vi "新版加标流程.vi"(8 "error in (no error)":errorcluster caption="错误输入（无错误）", 11 "参数":enum16{"氨氮", "总磷", "总氮", "CODMn", "CODcr"}(ring)) -> (0 "error out":errorcluster caption="错误输出")   [LabVIEW 2016, in "质控单元.lvlib"]
panel:
  out "Next State":string
  out "数值":i32
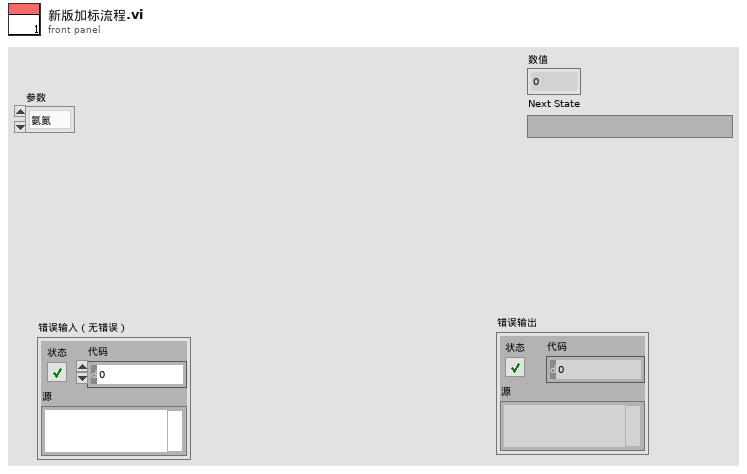
[diagram p1: front panel]
types:
  T1 = cluster{"时间标识":timestamp, "设备":string, "日志信息":string}
  T2 = enum16{"待机", "润洗中", "进样中", "加标中", "排液中", "搅拌中", "进样超时报警"}
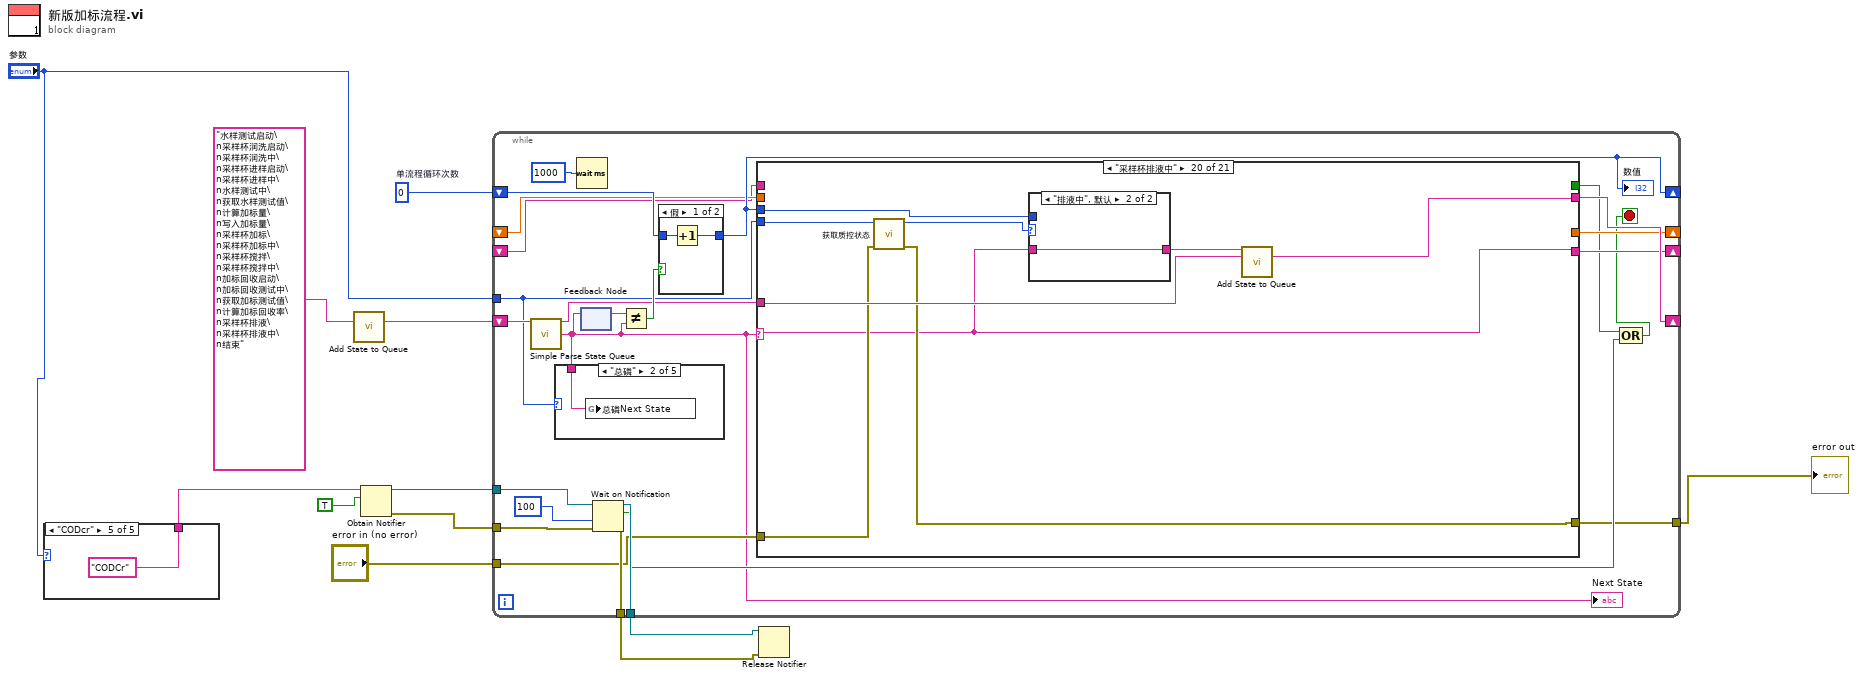
[diagram p0: block diagram]
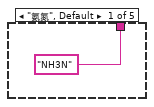
[diagram p2: hidden frame]
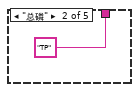
[diagram p3: hidden frame]
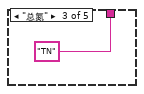
[diagram p4: hidden frame]
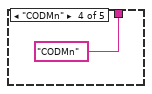
[diagram p5: hidden frame]
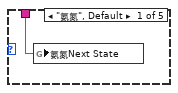
[diagram p6: hidden frame]
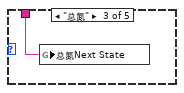
[diagram p7: hidden frame]
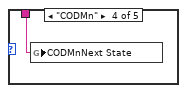
[diagram p8: hidden frame]
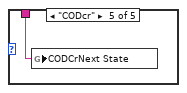
[diagram p9: hidden frame]
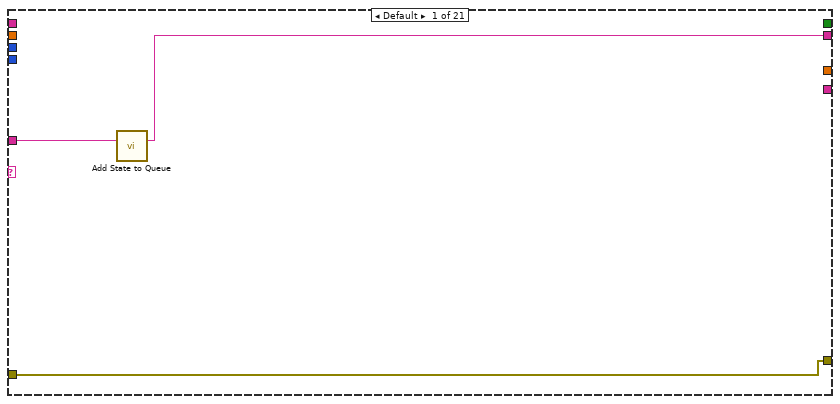
[diagram p11: hidden frame]
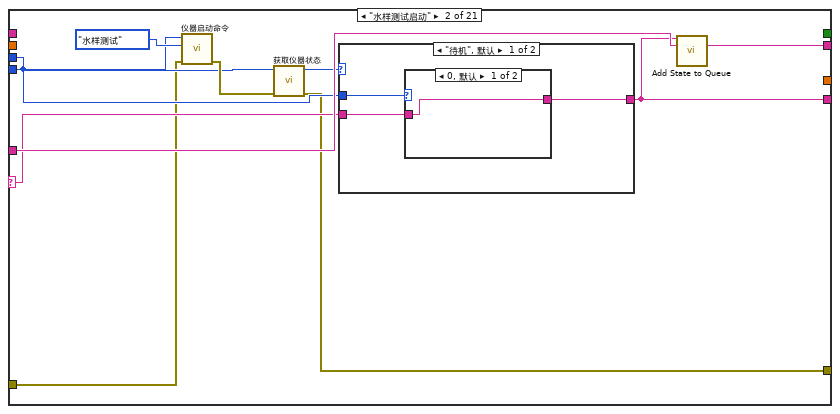
[diagram p12: hidden frame]
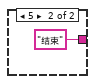
[diagram p13: hidden frame]
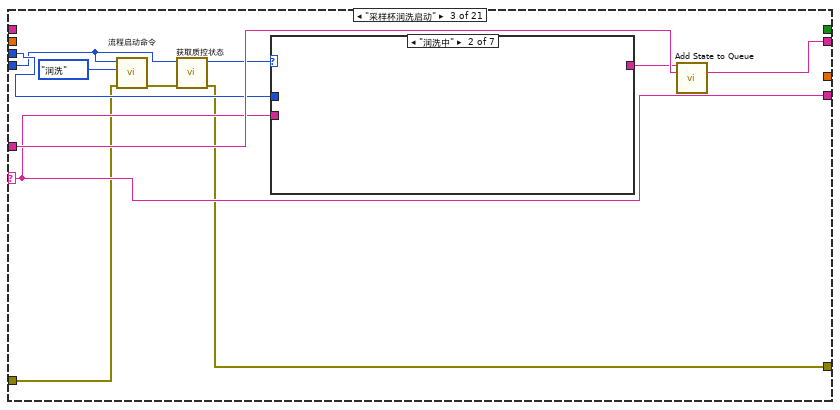
[diagram p15: hidden frame]
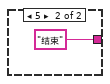
[diagram p17: hidden frame]
diagram:
  w10 = 0  # 单流程循环次数
  n1 = case shown="\"CODcr\"" "参数" {
    tunnel: ["NH3N" ("名称（未命名）") "TP" ("名称（未命名）") "TN" ("名称（未命名）") "CODMn" ("名称（未命名）") "CODCr" ("名称（未命名）")] -> w4
    frame "氨氮", Default {
    }
    frame "总磷" {
    }
    frame "总氮" {
    }
    frame "CODMn" {
    }
    frame "CODcr" {
    }
  }
  n2 = call "Add State to Queue.vi"("State(s) In (\"\")"="水样测试启动\n采样杯润洗启动\n采样杯润洗中\n采样杯进样启动\n采样杯进样中\n水样测试中\n获取水样测试值\n计算加标量\n写入加标量\n采样杯加标\n采样杯加标中\n采样杯搅拌\n采样杯搅拌中\n加标回收启动\n加标回收测试中\n获取加标测试值\n计算加标回收率\n采样杯排液\n采样杯排液中\n结束" ("State(s) In (\"\")")) -> ("States Out"=w11:string)  [unwired: 14 in]
  n3 = Obtain Notifier(name (unnamed)=w4, notification data type=TRUE) -> (notifier out=w6:refnum<notifier>, error out=w5:errorcluster)  [unwired: 2 in, 1 out]
  n4 = while {
    shift-right: [w40] -> _
    shift-left: w11 -> [w41]
    tunnel: "参数" -> [w19]
    shift-right: [w36] -> _
    shift-left: w10 -> [w37]
    shift-right: [w34] -> _
    shift-left: _ -> [w33]
    shift-right: [w32] -> _
    shift-left: _ -> [w31]
    tunnel: [w21] -> w8
    tunnel: "error in (no error)" -> [w20]
    tunnel: w6 -> [w29]
    tunnel: w5 -> [w28]
    tunnel: [w27] -> w2
    tunnel: [w26] -> w1
    stop <- w23 stop-if-true
    n5 = call "Simple Parse State Queue.vi"("State Queue"=w41) -> ("Remain States"=w22:string, "Next State"=w18:string)  [unwired: 13 in]
    "Next State" <- w18
    n6 = case shown="\"总磷\"" w19 {
      tunnel: w18 -> [w42 w43 w44 w45 w46]
      frame "氨氮", Default {
        n7 = global write "质控内部交互全局.vi" "氨氮Next State"(w42) -> ()
      }
      frame "总磷" {
        n8 = global write "质控内部交互全局.vi" "总磷Next State"(w43) -> ()
      }
      frame "总氮" {
        n9 = global write "质控内部交互全局.vi" "总氮Next State"(w44) -> ()
      }
      frame "CODMn" {
        n10 = global write "质控内部交互全局.vi" "CODMnNext State"(w45) -> ()
      }
      frame "CODcr" {
        n11 = global write "质控内部交互全局.vi" "CODCrNext State"(w46) -> ()
      }
    }
    n12 = Wait (ms)(milliseconds to wait=u32 1000 ("等待时间（毫秒）")) -> ()  [unwired: 1 out]
    n13 = feedback-in #1(w18) -> ()
    n14 = feedback #1() -> (w39:string)  [unwired: 1 in]
    n15 = Wait on Notification(notifier=w29, timeout in ms (-1)=100 ("超时毫秒(-1)"), error in (no error)=w28) -> (notifier out=w27:refnum<notifier>, notification=w24:bool, error out=w26:errorcluster)  [unwired: 1 in, 1 out]
    n16 = Not Equal?(x=w39, y=w18) -> (x != y?=w38:bool)
    n17 = case shown="假" w38 {
      tunnel: w37 -> [w48 _]
      tunnel: [w47 _] -> w36
      frame False {
        n18 = Increment(x=w48) -> (x+1=w47:i32)
      }
      frame True {
      }
    }
    "数值" <- w36
    n19 = case shown="\"采样杯排液中\"" w18 {
      selector: w18 -> [_ w56 w70 w88 w99 w115 w127 w136 w145 w159 w173 w185 w195 w207 w217 w233 w243 w254 w264 w277 w295]
      tunnel: w22 -> [w51 w61 w78 w93 w106 w121 w132 w141 w151 w165 w181 w191 w203 w211 w225 w239 w248 w257 w268 w281 w290]
      tunnel: [w50 w60 w77 w92 w105 w120 w131 w140 w150 w164 w180 w190 w202 w209 w224 w238 w247 w256 w265 w278 w297] -> w40
      tunnel: w19 -> [_ w58 w74 w90 w102 w117 w130 w139 w148 w162 w177 w188 w198 w210 w220 w237 w246 w252 w269 w282 w291]
      tunnel: w36 -> [_ w57 w76 w91 w104 w118 w129 w138 w149 w163 w179 w189 w201 w212 w223 w236 w245 w255 w270 w283 w296]
      tunnel: [_ _ _ _ _ _ _ _ _ _ _ _ _ _ _ _ _ _ _ _ TRUE] -> w25
      tunnel: [_ _ _ _ _ _ _ _ w147 _ _ _ _ _ _ _ _ _ _ _ _] -> w34
      tunnel: w33 -> [_ _ _ _ _ _ _ _ _ w161 _ _ _ _ _ _ _ _ _ _ _]
      tunnel: [_ w54 w70 w88 w99 w115 w127 w136 w145 w159 w173 w185 w195 w207 w217 w233 w243 w251 w264 w277 _] -> w32
      tunnel: w31 -> [_ _ _ _ _ _ _ _ _ _ _ _ _ _ _ _ _ _ _ _ w289]
      tunnel: [w49 w53 w69 w87 w97 w113 w125 w135 w143 w158 w172 w184 w194 w206 w216 w231 w242 w250 w266 w279 w286] -> w21
      tunnel: w20 -> [w49 w52 w68 w86 w96 w116 w124 w134 w144 w157 w171 w183 w193 w205 w215 w232 w241 w250 w267 w280 w286]
      frame Default {
        n20 = call "Add State to Queue.vi"("State(s) In (\"\")"=w51) -> ("States Out"=w50:string)  [unwired: 14 in]
      }
      frame "水样测试启动" {
        n21 = call "仪器启动命令.vi"("error in (no error)"=w52, "测试模式"=enum16{"水样测试", "加标回收"}."水样测试", "参数"=w58) -> ("error out"=w59:errorcluster)  [unwired: 8 in]
        n22 = call "获取仪器状态.vi"("error in (no error)"=w59, "参数"=w58) -> ("error out"=w53:errorcluster, "仪器状态"=w55:enum16{"待机", "运行"})  [unwired: 8 in]
        n23 = case shown="\"待机\", 默认" w55 {
          tunnel: w57 -> [w65 _]
          tunnel: w56 -> [w64 _]
          tunnel: [w63 _] -> w54
          frame "待机", Default {
            n24 = case shown="0, 默认" w65 {
              tunnel: w64 -> [w66 _]
              tunnel: [w66 "结束"] -> w63
              frame 0, Default {
              }
              frame 5 {
              }
            }
          }
          frame "运行" {
          }
        }
        n25 = call "Add State to Queue.vi"("State(s) In Front (\"\")"=w54, "State(s) In (\"\")"=w61) -> ("States Out"=w60:string)  [unwired: 13 in]
      }
      frame "采样杯润洗启动" {
        n26 = call "流程启动命令.vi"("error in (no error)"=w68, "流程"=enum16{"润洗", "进样", "加标", "搅拌", "排液"}."润洗", "参数"=w74) -> ("error out"=w72:errorcluster)  [unwired: 8 in]
        n27 = call "获取质控状态.vi"("error in (no error)"=w72, "参数"=w74) -> ("error out"=w69:errorcluster, "仪器状态"=w73:T2)  [unwired: 8 in]
        n28 = case shown="\"润洗中\"" w73 {
          tunnel: w76 -> [w81 _ _ _ _ _ _]
          tunnel: w70 -> [w80 _ _ _ _ _ _]
          tunnel: [w79 _ _ _ _ _ "结束"] -> w71
          frame "待机", Default {
            n29 = case shown="0, 默认" w81 {
              tunnel: w80 -> [w82 _]
              tunnel: [w82 "结束"] -> w79
              frame 0, Default {
              }
              frame 5 {
              }
            }
          }
          frame "润洗中" {
          }
          frame "进样中" {
          }
          frame "加标中" {
          }
          frame "排液中" {
          }
          frame "搅拌中" {
          }
          frame "进样超时报警" {
          }
        }
        n30 = call "Add State to Queue.vi"("State(s) In Front (\"\")"=w71, "State(s) In (\"\")"=w78) -> ("States Out"=w77:string)  [unwired: 13 in]
      }
      frame "采样杯润洗中" {
        n31 = call "获取质控状态.vi"("error in (no error)"=w86, "参数"=w90) -> ("error out"=w87:errorcluster, "仪器状态"=w85:T2)  [unwired: 8 in]
        n32 = case shown="\"润洗中\", 默认" w85 {
          tunnel: w91 -> [_ _ _]
          tunnel: w88 -> [_ w94 _]
          tunnel: [_ w94 "结束"] -> w89
          frame "待机" {
          }
          frame "润洗中", Default {
          }
          frame "进样超时报警" {
          }
        }
        n33 = call "Add State to Queue.vi"("State(s) In Front (\"\")"=w89, "State(s) In (\"\")"=w93) -> ("States Out"=w92:string)  [unwired: 13 in]
      }
      frame "采样杯进样启动" {
        n34 = call "流程启动命令.vi"("error in (no error)"=w96, "流程"=enum16{"润洗", "进样", "加标", "搅拌", "排液"}."进样", "参数"=w102) -> ("error out"=w98:errorcluster)  [unwired: 8 in]
        n35 = call "获取质控状态.vi"("error in (no error)"=w98, "参数"=w102) -> ("error out"=w97:errorcluster, "仪器状态"=w101:T2)  [unwired: 8 in]
        n36 = case shown="\"待机\", 默认" w101 {
          tunnel: w104 -> [w109 _ _]
          tunnel: w99 -> [w108 _ _]
          tunnel: [w107 _ "结束"] -> w100
          frame "待机", Default {
            n37 = case shown="0, 默认" w109 {
              tunnel: w108 -> [w110 _]
              tunnel: [w110 "结束"] -> w107
              frame 0, Default {
              }
              frame 5 {
              }
            }
          }
          frame "进样中" {
          }
          frame "进样超时报警" {
          }
        }
        n38 = call "Add State to Queue.vi"("State(s) In Front (\"\")"=w100, "State(s) In (\"\")"=w106) -> ("States Out"=w105:string)  [unwired: 13 in]
      }
      frame "采样杯进样中" {
        n39 = call "获取质控状态.vi"("error in (no error)"=w116, "参数"=w117) -> ("error out"=w113:errorcluster, "仪器状态"=w119:T2)  [unwired: 8 in]
        n40 = case shown="\"进样中\", 默认" w119 {
          tunnel: w118 -> [_ _ _]
          tunnel: w115 -> [_ w122 _]
          tunnel: [_ w122 "结束"] -> w114
          frame "待机" {
          }
          frame "进样中", Default {
          }
          frame "进样超时报警" {
          }
        }
        n41 = call "Add State to Queue.vi"("State(s) In Front (\"\")"=w114, "State(s) In (\"\")"=w121) -> ("States Out"=w120:string)  [unwired: 13 in]
      }
      frame "水样测试中" {
        n42 = call "获取仪器状态.vi"("error in (no error)"=w124, "参数"=w130) -> ("error out"=w125:errorcluster, "仪器状态"=w128:enum16{"待机", "运行"})  [unwired: 8 in]
        n43 = case shown="\"待机\"" w128 {
          tunnel: w129 -> [_ _]
          tunnel: w127 -> [_ w133]
          tunnel: [_ w133] -> w126
          frame "待机" {
          }
          frame "运行", Default {
          }
        }
        n44 = call "Add State to Queue.vi"("State(s) In Front (\"\")"=w126, "State(s) In (\"\")"=w132) -> ("States Out"=w131:string)  [unwired: 13 in]
      }
      frame "获取水样测试值" {
        n45 = call "获取仪器状态.vi"("error in (no error)"=w134, "参数"=w139) -> ("error out"=w135:errorcluster)  [unwired: 8 in, 1 out]
        n46 = case shown="0, 默认" w138 {
          tunnel: w136 -> [w142 _]
          tunnel: [w142 _] -> w137
          frame 0, Default {
          }
          frame 5 {
          }
        }
        n47 = call "Add State to Queue.vi"("State(s) In Front (\"\")"=w137, "State(s) In (\"\")"=w141) -> ("States Out"=w140:string)  [unwired: 13 in]
      }
      frame "计算加标量" {
        n48 = call "计算加标体积.vi"("error in (no error)"=w144, "参数"=w148) -> ("error out"=w143:errorcluster, "加标体积"=w147:dbl)  [unwired: 7 in, 1 out]
        n49 = case shown="错误" w143 {
          tunnel: w149 -> [_ w154]
          tunnel: w145 -> [_ w153]
          tunnel: [_ w152] -> w146
          frame No Error {
          }
          frame Error {
            n50 = case shown="5" w154 {
              tunnel: w153 -> [w155 _]
              tunnel: [w155 "结束"] -> w152
              frame 0, Default {
              }
              frame 5 {
              }
            }
          }
        }
        n51 = call "Add State to Queue.vi"("State(s) In Front (\"\")"=w146, "State(s) In (\"\")"=w151) -> ("States Out"=w150:string)  [unwired: 13 in]
      }
      frame "写入加标量" {
        n52 = call "写入加标体积.vi"("加标体积"=w161, "error in (no error)"=w157, "参数"=w162) -> ("error out"=w158:errorcluster)  [unwired: 8 in]
        n53 = case shown="错误" w158 {
          tunnel: w163 -> [_ w168]
          tunnel: w159 -> [_ w167]
          tunnel: [_ w166] -> w160
          frame No Error {
          }
          frame Error {
            n54 = case shown="5" w168 {
              tunnel: w167 -> [w169 _]
              tunnel: [w169 "结束"] -> w166
              frame 0, Default {
              }
              frame 5 {
              }
            }
          }
        }
        n55 = call "Add State to Queue.vi"("State(s) In Front (\"\")"=w160, "State(s) In (\"\")"=w165) -> ("States Out"=w164:string)  [unwired: 13 in]
      }
      frame "采样杯加标" {
        n56 = call "流程启动命令.vi"("error in (no error)"=w171, "流程"=enum16{"润洗", "进样", "加标", "搅拌", "排液"}."加标", "参数"=w177) -> ("error out"=w176:errorcluster)  [unwired: 8 in]
        n57 = call "获取质控状态.vi"("error in (no error)"=w176, "参数"=w177) -> ("error out"=w172:errorcluster, "仪器状态"=w175:T2)  [unwired: 8 in]
        n58 = case shown="\"待机\", 默认" w175 {
          tunnel: w179 -> [_ _]
          tunnel: w173 -> [w182 _]
          tunnel: [w182 _] -> w174
          frame "待机", Default {
          }
          frame "加标中" {
          }
        }
        n59 = call "Add State to Queue.vi"("State(s) In Front (\"\")"=w174, "State(s) In (\"\")"=w181) -> ("States Out"=w180:string)  [unwired: 13 in]
      }
      frame "采样杯加标中" {
        n60 = call "获取质控状态.vi"("error in (no error)"=w183, "参数"=w188) -> ("error out"=w184:errorcluster, "仪器状态"=w187:T2)  [unwired: 8 in]
        n61 = case shown="\"加标中\", 默认" w187 {
          tunnel: w189 -> [_ _]
          tunnel: w185 -> [_ w192]
          tunnel: [_ w192] -> w186
          frame "待机" {
          }
          frame "加标中", Default {
          }
        }
        n62 = call "Add State to Queue.vi"("State(s) In Front (\"\")"=w186, "State(s) In (\"\")"=w191) -> ("States Out"=w190:string)  [unwired: 13 in]
      }
      frame "采样杯搅拌" {
        n63 = call "流程启动命令.vi"("error in (no error)"=w193, "流程"=enum16{"润洗", "进样", "加标", "搅拌", "排液"}."搅拌", "参数"=w198) -> ("error out"=w199:errorcluster)  [unwired: 8 in]
        n64 = call "获取质控状态.vi"("error in (no error)"=w199, "参数"=w198) -> ("error out"=w194:errorcluster, "仪器状态"=w197:T2)  [unwired: 8 in]
        n65 = case shown="\"搅拌中\"" w197 {
          tunnel: w201 -> [_ _]
          tunnel: w195 -> [w204 _]
          tunnel: [w204 _] -> w196
          frame "待机", Default {
          }
          frame "搅拌中" {
          }
        }
        n66 = call "Add State to Queue.vi"("State(s) In Front (\"\")"=w196, "State(s) In (\"\")"=w203) -> ("States Out"=w202:string)  [unwired: 13 in]
      }
      frame "采样杯搅拌中" {
        n67 = call "获取质控状态.vi"("error in (no error)"=w205, "参数"=w210) -> ("error out"=w206:errorcluster, "仪器状态"=w213:T2)  [unwired: 8 in]
        n68 = case shown="\"搅拌中\", 默认" w213 {
          tunnel: w212 -> [_ _]
          tunnel: w207 -> [_ w214]
          tunnel: [_ w214] -> w208
          frame "待机" {
          }
          frame "搅拌中", Default {
          }
        }
        n69 = call "Add State to Queue.vi"("State(s) In Front (\"\")"=w208, "State(s) In (\"\")"=w211) -> ("States Out"=w209:string)  [unwired: 13 in]
      }
      frame "加标回收启动" {
        n70 = call "仪器启动命令.vi"("error in (no error)"=w215, "测试模式"=enum16{"水样测试", "加标回收"}."加标回收", "参数"=w220) -> ("error out"=w221:errorcluster)  [unwired: 8 in]
        n71 = call "获取仪器状态.vi"("error in (no error)"=w221, "参数"=w220) -> ("error out"=w216:errorcluster, "仪器状态"=w219:enum16{"待机", "运行"})  [unwired: 8 in]
        n72 = case shown="\"待机\", 默认" w219 {
          tunnel: w223 -> [w228 _]
          tunnel: w217 -> [w227 _]
          tunnel: [w226 _] -> w218
          frame "待机", Default {
            n73 = case shown="5" w228 {
              tunnel: w227 -> [w229 _]
              tunnel: [w229 "结束"] -> w226
              frame 0, Default {
              }
              frame 5 {
              }
            }
          }
          frame "运行" {
          }
        }
        n74 = call "Add State to Queue.vi"("State(s) In Front (\"\")"=w218, "State(s) In (\"\")"=w225) -> ("States Out"=w224:string)  [unwired: 13 in]
      }
      frame "加标回收测试中" {
        n75 = call "获取仪器状态.vi"("error in (no error)"=w232, "参数"=w237) -> ("error out"=w231:errorcluster, "仪器状态"=w235:enum16{"待机", "运行"})  [unwired: 8 in]
        n76 = case shown="\"运行\"" w235 {
          tunnel: w236 -> [_ _]
          tunnel: w233 -> [_ w240]
          tunnel: [_ w240] -> w234
          frame "待机", Default {
          }
          frame "运行" {
          }
        }
        n77 = call "Add State to Queue.vi"("State(s) In Front (\"\")"=w234, "State(s) In (\"\")"=w239) -> ("States Out"=w238:string)  [unwired: 13 in]
      }
      frame "获取加标测试值" {
        n78 = call "获取仪器状态.vi"("error in (no error)"=w241, "参数"=w246) -> ("error out"=w242:errorcluster)  [unwired: 8 in, 1 out]
        n79 = case shown="0, 默认" w245 {
          tunnel: w243 -> [w249 _]
          tunnel: [w249 _] -> w244
          frame 0, Default {
          }
          frame 5 {
          }
        }
        n80 = call "Add State to Queue.vi"("State(s) In Front (\"\")"=w244, "State(s) In (\"\")"=w248) -> ("States Out"=w247:string)  [unwired: 13 in]
      }
      frame "计算加标回收率" {
        n81 = case shown="5" w255 {
          tunnel: w254 -> [w263 _]
          tunnel: [w263 _] -> w251
          frame 0, Default {
          }
          frame 5 {
          }
        }
        n82 = case shown="\"总磷\"" w252 {
          tunnel: TRUE ("氨氮加标回收测完标志") -> [w258 w259 w260 w261 w262]
          frame "氨氮", Default {
            n83 = global write "质控测完标志全局 1.vi" "氨氮加标回收测完标志"(w258) -> ()
          }
          frame "总磷" {
            n84 = global write "质控测完标志全局 1.vi" "总磷加标回收测完标志"(w259) -> ()
          }
          frame "总氮" {
            n85 = global write "质控测完标志全局 1.vi" "总氮加标回收测完标志"(w260) -> ()
          }
          frame "CODMn" {
            n86 = global write "质控测完标志全局 1.vi" "COD加标回收测完标志"(w261) -> ()
          }
          frame "CODcr" {
            n87 = global write "质控测完标志全局 1.vi" "CODCr加标回收测完标志"(w262) -> ()
          }
        }
        n88 = call "Add State to Queue.vi"("State(s) In Front (\"\")"=w251, "State(s) In (\"\")"=w257) -> ("States Out"=w256:string)  [unwired: 13 in]
      }
      frame "采样杯排液" {
        n89 = call "流程启动命令.vi"("error in (no error)"=w267, "流程"=enum16{"润洗", "进样", "加标", "搅拌", "排液"}."排液", "参数"=w269) -> ("error out"=w273:errorcluster)  [unwired: 8 in]
        n90 = call "获取质控状态.vi"("error in (no error)"=w273, "参数"=w269) -> ("error out"=w266:errorcluster, "仪器状态"=w272:T2)  [unwired: 8 in]
        n91 = case shown="\"排液中\"" w272 {
          tunnel: w270 -> [_ _]
          tunnel: w264 -> [w275 _]
          tunnel: [w275 _] -> w271
          frame "待机", Default {
          }
          frame "排液中" {
          }
        }
        n92 = call "Add State to Queue.vi"("State(s) In Front (\"\")"=w271, "State(s) In (\"\")"=w268) -> ("States Out"=w265:string)  [unwired: 13 in]
      }
      frame "采样杯排液中" {
        n93 = call "获取质控状态.vi"("error in (no error)"=w280, "参数"=w282) -> ("error out"=w279:errorcluster, "仪器状态"=w276:T2)  [unwired: 8 in]
        n94 = case shown="\"排液中\", 默认" w276 {
          tunnel: w283 -> [_ _]
          tunnel: w277 -> [_ w285]
          tunnel: [_ w285] -> w284
          frame "待机" {
          }
          frame "排液中", Default {
          }
        }
        n95 = call "Add State to Queue.vi"("State(s) In Front (\"\")"=w284, "State(s) In (\"\")"=w281) -> ("States Out"=w278:string)  [unwired: 13 in]
      }
      frame "结束" {
        n96 = call "获取仪器状态.vi"("参数"=w291) -> ()  [unwired: 9 in, 2 out]
        n97 = case shown="0, 默认" w296 {
          tunnel: w295 -> [w310 _]
          tunnel: [w310 _] -> w294
          frame 0, Default {
          }
          frame 5 {
          }
        }
        n98 = case shown="\"氨氮\", 默认" w291 {
          tunnel: FALSE ("氨氮加标回收测完标志") -> [w305 w306 w307 w308 w309]
          frame "氨氮", Default {
            n99 = global write "质控测完标志全局 1.vi" "氨氮加标回收测完标志"(w305) -> ()
          }
          frame "总磷" {
            n100 = global write "质控测完标志全局 1.vi" "总磷加标回收测完标志"(w306) -> ()
          }
          frame "总氮" {
            n101 = global write "质控测完标志全局 1.vi" "总氮加标回收测完标志"(w307) -> ()
          }
          frame "CODMn" {
            n102 = global write "质控测完标志全局 1.vi" "COD加标回收测完标志"(w308) -> ()
          }
          frame "CODcr" {
            n103 = global write "质控测完标志全局 1.vi" "CODCr加标回收测完标志"(w309) -> ()
          }
        }
        n104 = Equal?(x=w289, y="结束") -> (x = y?=w287:bool)
        n105 = case shown="真" w287 {
          tunnel: w289 -> [w304 _]
          frame False {
            n106 = Concatenate Strings(w304, "失败" ("字符串")) -> (w298:string)
            n107 = Get Date/Time In Seconds() -> (seconds since 1Jan1904=w302:timestamp)
            n108 = Bundle By Name(cluster=T1 {"时间标识"=timestamp(0 s since 1904-01-01), "设备"="", "日志信息"=""} ("data in"), "时间标识"=w302, "设备"="质控单元", "日志信息"=w298) -> (w299:T1)
            n109 = call "质控报警信息.vi"("data in"=w299) -> ()  [unwired: 11 in]
          }
          frame True {
            (unwired) ""
          }
        }
        n110 = call "Add State to Queue.vi"("State(s) In Front (\"\")"=w294, "State(s) In (\"\")"=w290) -> ("States Out"=w297:string)  [unwired: 13 in]
      }
    }
    n111 = Compound Arithmetic op=OR ("复合运算")(w25, w24) -> (w23:bool)
  }
  "error out" <- w8
  n112 = Release Notifier(notifier=w2, error in (no error)=w1) -> ()  [unwired: 1 in, 3 out]
